vi "Demo.vi"() -> ()   [LabVIEW 2011, in "Image Converter.lvlib"]
uses:
  Image Converter.lvlib
panel:
  in  "Output Image Type":T1(ring)
  in  "Image Save Path":path
  in  "Image Input Path":path
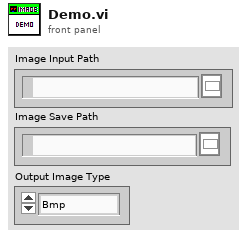
[diagram p1: front panel]
types:
  T1 = enum16{"Bmp", "Emf", "Exif", "Gif", "Icon", "Jpeg", "MemoryBmp", "Png", "Tiff", "Wmf"}
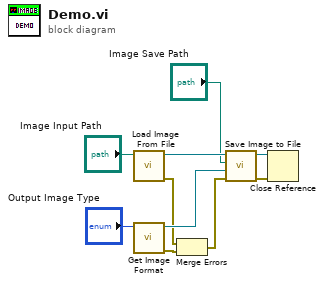
[diagram p0: block diagram]
diagram:
  n1 = call "Load Image From File.vi"("Image Input Path"="Image Input Path") -> ("错误输出"=w4:errorcluster, "FromFile"=w9:refnum<k24>)  [unwired: 9 in]
  n2 = call "Get Image Format.vi"("Output Image Type"="Output Image Type") -> ("错误输出"=w3:errorcluster, "Image Format"=w8:refnum<k24>)  [unwired: 9 in]
  n3 = Merge Errors(w4, w3) -> (w2:errorcluster)
  n4 = call "Save Image to File.vi"("错误输入（无错误）"=w2, "Image Format"=w8, "Image Save Path"="Image Save Path", "Image Ref In"=w9) -> ("错误输出"=w5:errorcluster, "Image Ref Out"=w6:refnum<k24>)  [unwired: 6 in]
  n5 = Close Reference(reference=w6, error in (no error)=w5) -> ()  [unwired: 1 out]
